vi "dfd_Get Zeros in the Upper Half Plane.vi"(8 "error in (no error)":errorcluster, 11 "zeros":cdb[](array[numeric])) -> (0 "error out":errorcluster, 2 "half zeros":cdb[](array[numeric]))   [LabVIEW 2017, in "NI_DigFilter_Design.lvlib"]
uses:
  <vilib>/addons/Digital Filter Design/NI_DigFilter_Design.lvlib
  <vilib>/addons/Digital Filter Design/_Misc.llb/dfd_Error Cluster From Error Code (Scalar).vi
  <vilib>/Analysis/NI_AALPro.lvlib
  <vilib>/addons/Digital Filter Design/NI_DigFilterLicensed.lvlib
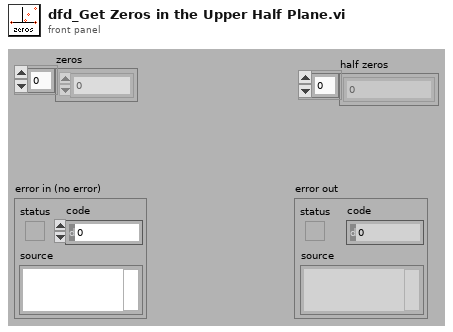
[diagram p1: front panel]
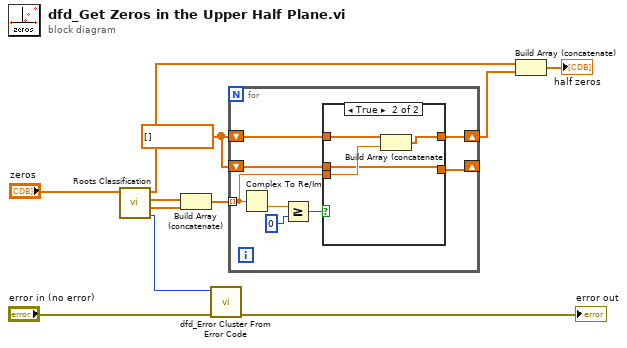
[diagram p0: block diagram]
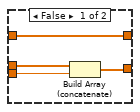
[diagram p2: hidden frame]
diagram:
  w7 = cdb[] []
  n1 = call <vilib>:"Roots Classification.vi"("Roots"="zeros") -> ("error"=w2:i32, "Pure Complex Roots"=w9:cdb[], "Complex Pair Roots"=w10:cdb[], "Real Roots"=w11:dbl[])  [unwired: 2 in, 5 out]
  n2 = Build Array (concatenate)(w10, w9) -> (w8:cdb[])
  n3 = call-poly <vilib>:"dfd_Error Cluster From Error Code.vi"("error in (no error)"="error in (no error)", "error code (0)"=w2) -> ("error out"=→"error out":errorcluster)  [unwired: 9 out]
  n4 = for {
    tunnel: w8 -> [w15] mode=indexing
    shift-right: [w16] -> w6
    shift-left: w7 -> [w14]
    shift-right: [w12] -> _
    shift-left: w7 -> [w13]
    n5 = Complex To Re/Im(x + iy=w15) -> (y=w19:dbl)  [unwired: 1 out]
    n6 = Greater Or Equal?(x=w19, y=0) -> (x >= y?=w17:bool)
    n7 = case shown="True" w17 {
      tunnel: [w20 w27] -> w16
      tunnel: w15 -> [w22 w26]
      tunnel: w14 -> [w20 w25]
      tunnel: [w21 w24] -> w12
      tunnel: w13 -> [w23 w24]
      frame False {
        n8 = Build Array (concatenate)(w23, w22) -> (w21:cdb[])
      }
      frame True {
        n9 = Build Array (concatenate)(w25, w26) -> (w27:cdb[])
      }
    }
  }
  n10 = Build Array (concatenate)(w11, w6) -> (→"half zeros":cdb[])
